vi "Send_JSN_Message_2 (SubVI).vi"(6 "id":i32, 9 "data":cluster{"name":string, "value":T1}={"name"="i_range", "value"=enum."auto"}, 11 "type":string="start") -> (2 "JSON message":string)   [LabVIEW 2015]
uses:
  Ctrl/I_range.ctl
  Ctrl/R_W.ctl
  JSON_conv/Conv_JSON_6 (SubVI).vi
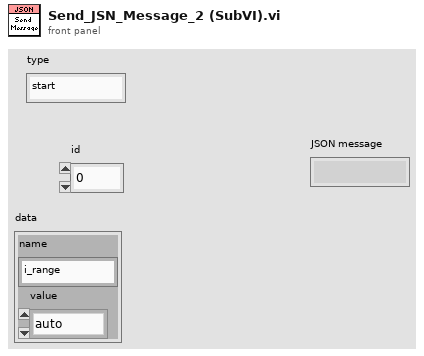
[diagram p1: front panel]
types:
  T1 = typedef "I_range.ctl" = enum16{"off", "18 µA", "180 µA", "1.8 mA", "18 mA", "180 mA", "2 A", "10 A", "auto"}
  T2 = cluster{"type":string, "phase":string, "id":u8, "status":i32, "status_msg":string, "device":string}
  T3 = typedef "R_W.ctl" = enum16{"Write", "Read", "RAZ"}
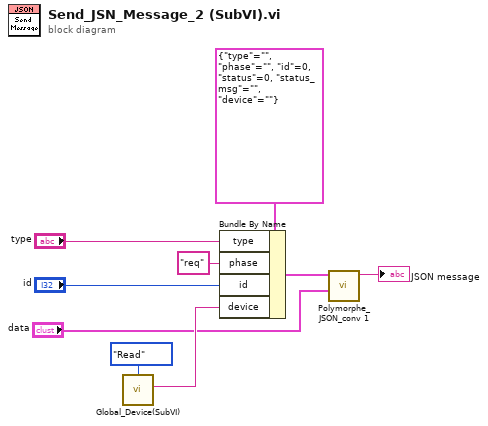
[diagram p0: block diagram]
diagram:
  n1 = call "Global_Device(SubVI).vi"("R/W"=R_W."Read") -> ("Device out"=w9:string)  [unwired: 10 in]
  n2 = Bundle By Name(cluster=T2 {"type"="", "phase"="", "id"=0, "status"=0, "status_msg"="", "device"=""}, "type"="type", "phase"="req", "id"="id", "device"=w9) -> (w4:T2)
  n3 = call-poly "Polymorphe_JSON_conv 1.vi"("data"="data", "Cluster"=w4) -> ("String"=→"JSON message":string)  [unwired: 9 in]
